vi "realtime track laser dot.vi"() -> ()   [LabVIEW 2015]
doc: "The Low-Level Grab VI acquires images continuously and displays the images in an image control using low-level acquisition VIs. A grab is appropriate for high-speed applications in which you need to process only one image at a time."
uses:
  <vilib>/userdefined/High Color/IMAQdx.ctl
  <vilib>/vision/driver/IMAQdx.llb/IMAQdx Buffer Number Mode.ctl
  <vilib>/vision/driver/NI_Vision_Acquisition_Software.lvlib
  <resource>/objmgr/imaqdx.rc
panel:
  in  "Color of Overlay Text":u32(colorbox)=16448250
  out "time vs iteration":cluster{dbl[], i32[]}(graph)
  out "FPS":i32=42
  out "time (s)":dbl[](array[numeric])=[0.0, 0.04, 0.066, 0.087, 0.114, 0.136, 0.161, 0.184, 0.208, 0.232, 0.257, 0.278, 0.305, 0.328, 0.352, 0.378, 0.399, 0.424, 0.448, 0.473, 0.497, 0.521, 0.545, 0.572, 0.59, 0.614, 0.639, 0.662, 0.686, 0.712, 0.736, 0.761, 0.787, 0.809, 0.834, 0.858, 0.881, 0.907, 0.928, 0.952, 0.978, 1.002, 1.028, 1.049, 1.075, 1.098, 1.124, 1.146, 1.171, 1.197, 1.218, 1.241, 1.267, 1.304, 1.317, 1.336, 1.364, 1.399, 1.411, 1.435, 1.464, 1.49, 1.504, 1.528, 1.566, 1.578, 1.608, 1.629, 1.664, 1.678, 1.709, 1.722, 1.745, 1.768, 1.794, 1.817, 1.842, 1.865, 1.888, 1.913, 1.937, 1.962, 1.987, 2.01, 2.033, 2.058, 2.082, 2.107, 2.132, 2.156, 2.179, 2.203, 2.229, 2.252, 2.278, 2.3, 2.323, 2.348, 2.372, 2.414, 2.426, 2.45, 2.465, 2.489, 2.513, 2.538, 2.562, 2.586, 2.611, 2.634, 2.659, 2.682, 2.708, 2.73, 2.754, 2.778, 2.802, 2.827, 2.85, 2.874, 2.898, 2.922, 2.945, 2.97, 2.995, 3.018, 3.042, 3.066, 3.09, 3.116, 3.139, 3.162, 3.186, 3.211, 3.233, 3.259, 3.282, 3.307, 3.33, 3.355, 3.379, 3.402, 3.427, 3.45, 3.475, 3.499, 3.524, 3.546, 3.571, 3.594, 3.619, 3.643, 3.666, 3.691, 3.715, 3.739, 3.763, 3.787, 3.811, 3.834, 3.86, 3.883, 3.908, 3.931, 3.956, 3.979, 4.003, 4.028, 4.05, 4.076, 4.099, 4.124, 4.147, 4.172, 4.195, 4.219, 4.244, 4.267, 4.292, 4.315, 4.34, 4.363, 4.388, 4.412, 4.437, 4.46, 4.483, 4.51, 4.534, 4.556, 4.582, 4.604, 4.629, 4.653, 4.677, 4.7, 4.725, 4.748, 4.772, 4.796, 4.82, 4.847, 4.868, 4.893, 4.917, 4.941, 4.965, 4.989, 5.013, 5.038, 5.061, 5.085, 5.111, 5.133, 5.159, 5.181, 5.205, 5.229, 5.253, 5.278, 5.301, 5.326, 5.349, 5.374, 5.398, 5.422, 5.445, 5.47, 5.494, 5.518, 5.541, 5.567, 5.59, 5.614, 5.638, 5.662, 5.686, 5.71, 5.734, 5.759, 5.782, 5.806, 5.834, 5.854, 5.879, 5.903, 5.927, 5.95, 5.976, 5.999, 6.023, 6.047, 6.072, 6.095, 6.121, 6.144, 6.167, 6.192, 6.215, 6.24, 6.263, 6.288, 6.312, 6.336, 6.36, 6.383, 6.408, 6.432, 6.457, 6.48, 6.505, 6.529, 6.552, 6.577, 6.6, 6.626, 6.648, 6.673, 6.696, 6.721, 6.746, 6.768, 6.794, 6.816, 6.843, 6.865, 6.89, 6.913, 6.938, 6.962, 6.985, 7.01, 7.034, 7.058, 7.082, 7.106, 7.13, 7.154, 7.178, 7.202, 7.227, 7.25, 7.274, 7.298, 7.322, 7.346, 7.37, 7.395, 7.418, 7.443, 7.466, 7.491, 7.514, 7.539, 7.562, 7.586, 7.611, 7.634, 7.66, 7.682, 7.708, 7.73, 7.756, 7.779, 7.804, 7.827, 7.851, 7.876, 7.899, 7.924, 7.947, 7.971, 7.995, 8.019, 8.043, 8.067, 8.092, 8.116, 8.14, 8.163, 8.187, 8.212, 8.235, 8.26, 8.283, 8.309, 8.331, 8.356, 8.379, 8.404, 8.428, 8.452, 8.477, 8.5, 8.524, 8.551, 8.575, 8.597, 8.621, 8.645, 8.668, 8.694, 8.717, 8.743, 8.765, 8.79, 8.812, 8.837, 8.862, 8.888, 8.913, 8.936, 8.959, 8.986, 9.009, 9.033, 9.057, 9.082, 9.11, 9.128, 9.151, 9.175, 9.202, 9.228, 9.248, 9.271, 9.295, 9.319, 9.344, 9.384, 9.397, 9.415, 9.441, 9.478, 9.491, 9.521, 9.536, 9.563, 9.584, 9.609, 9.631, 9.67, 9.683, 9.706, 9.729, 9.752, 9.776, 9.812, 9.826, 9.849, 9.881, 9.899, 9.922, 9.944, 9.969, 9.993, 10.016, 10.041, 10.066, 10.091, 10.118, 10.14, 10.165, 10.184, 10.21, 10.234, 10.258, 10.294, 10.308, 10.342, 10.355, 10.377, 10.411, 10.424, 10.449, 10.475, 10.507, 10.523, 10.549, 10.58, 10.595, 10.618, 10.646, 10.668, 10.693, 10.716, 10.739, 10.762, 10.8, 10.813, 10.837, 10.862, 10.9, 10.913, 10.931, 10.955, 10.981, 11.007, 11.044, 11.058, 11.076, 11.103, 11.128, 11.15, 11.175, 11.197, 11.23, 11.245, 11.271, 11.294, 11.319, 11.342, 11.37, 11.39, 11.417, 11.438, 11.465, 11.486, 11.512, 11.532, 11.557, 11.581, 11.605, 11.638, 11.654, 11.68, 11.701, 11.727, 11.768, 11.782, 11.797, 11.822, 11.847, 11.873, 11.895, 11.92, 11.943, 11.97, 11.991, 12.016, 12.04, 12.064, 12.099, 12.113, 12.138, 12.159, 12.183, 12.208, 12.234, 12.257, 12.287, 12.309, 12.328, 12.355, 12.375, 12.399, 12.424, 12.451, 12.471, 12.495, 12.519, 12.565, 12.579, 12.592, 12.616, 12.643, 12.661, 12.708, 12.724, 12.736, 12.76, 12.784, 12.81, 12.832, 12.858, 12.88, 12.904, 12.929, 12.952, 12.979, 13.0, 13.025, 13.051, 13.073, 13.098, 13.127, 13.145, 13.169, 13.194, 13.219, 13.241, 13.268, 13.287, 13.313, 13.34, 13.361, 13.388, 13.408, 13.432, 13.459, 13.481, 13.507, 13.529, 13.554, 13.581, 13.602, 13.629, 13.65, 13.676, 13.699, 13.727, 13.747, 13.775, 13.794, 13.819, 13.844, 13.867, 13.893, 13.915, 13.94, 13.965, 13.988, 14.01, 14.04, 14.057, 14.082, 14.108, 14.133, 14.156, 14.18, 14.205, 14.232, 14.252, 14.278, 14.3, 14.326, 14.348, 14.373, 14.397, 14.421, 14.446, 14.468, 14.494, 14.516, 14.541, 14.565, 14.59, 14.611, 14.639, 14.66, 14.688, 14.708, 14.736, 14.757, 14.785, 14.804, 14.83, 14.853, 14.877, 14.902, 14.926, 14.948, 14.974, 14.995, 15.02, 15.046, 15.071, 15.095, 15.121, 15.142, 15.169, 15.191, 15.216, 15.237, 15.263, 15.287, 15.311, 15.333, 15.359, 15.382, 15.409, 15.431, 15.454, 15.48, 15.502, 15.528, 15.55, 15.575, 15.6, 15.621, 15.646, 15.674, 15.696, 15.716, 15.744, 15.768, 15.792, 15.817, 15.84, 15.864, 15.887, 15.912, 15.934, 15.962, 15.984, 16.007, 16.036, 16.056, 16.081, 16.105, 16.129, 16.153, 16.176, 16.2, 16.229, 16.249, 16.273, 16.298, 16.319, 16.348, 16.369, 16.392, 16.419, 16.441, 16.464, 16.492, 16.512, 16.542, 16.56, 16.586, 16.608, 16.633, 16.659, 16.679, 16.704, 16.732, 16.751, 16.777, 16.8, 16.826, 16.848, 16.875, 16.896, 16.92, 16.946, 16.969, 16.995, 17.017, 17.042, 17.063, 17.089, 17.117, 17.139, 17.162, 17.184, 17.211, 17.233, 17.26, 17.281, 17.307, 17.329, 17.357, 17.376, 17.401, 17.426, 17.451, 17.473, 17.499, 17.522, 17.546, 17.573, 17.593, 17.619, 17.642, 17.668, 17.691, 17.713, 17.738, 17.763, 17.792, 17.812, 17.834, 17.861, 17.886, 17.908, 17.933, 17.956, 17.98, 18.005, 18.029, 18.051, 18.078, 18.1, 18.125, 18.15, 18.175, 18.196, 18.221, 18.245, 18.269, 18.293, 18.319, 18.342, 18.366, 18.39, 18.414, 18.438, 18.462, 18.486, 18.511, 18.534, 18.558, 18.583, 18.606, 18.628, 18.657, 18.676, 18.702, 18.724, 18.754, 18.772, 18.797, 18.822, 18.845, 18.867, 18.895, 18.918, 18.941, 18.967, 18.991, 19.013, 19.039, 19.062, 19.085, 19.114, 19.136, 19.158, 19.182, 19.205, 19.229, 19.255, 19.279, 19.303, 19.326, 19.349, 19.376, 19.398, 19.425, 19.444, 19.472, 19.494, 19.52, 19.542, 19.568, 19.591, 19.615, 19.639, 19.663, 19.686, 19.715, 19.733, 19.761, 19.782, 19.809, 19.83, 19.856, 19.877, 19.905, 19.926, 19.951, 19.975, 20.005, 20.023, 20.048, 20.07, 20.096, 20.136, 20.153, 20.168, 20.193, 20.218, 20.24, 20.264, 20.286, 20.322, 20.336, 20.364, 20.385, 20.41, 20.433, 20.456, 20.48, 20.507, 20.529, 20.553, 20.579, 20.601, 20.626, 20.649, 20.673, 20.699, 20.721, 20.745, 20.769, 20.793, 20.824, 20.845, 20.871, 20.887, 20.915, 20.939, 20.962, 20.984, 21.012, 21.037, 21.058, 21.083, 21.106, 21.133, 21.155, 21.181, 21.205, 21.23, 21.252, 21.276, 21.301, 21.324, 21.348, 21.373, 21.396, 21.42, 21.444, 21.47, 21.492, 21.516, 21.54, 21.565, 21.589, 21.612, 21.636, 21.66, 21.687, 21.71, 21.736, 21.758, 21.783, 21.806, 21.832, 21.856, 21.879, 21.903, 21.926, 21.951, 21.975, 22.003, 22.024, 22.047, 22.072, 22.096, 22.123, 22.143, 22.167, 22.188, 22.213, 22.239, 22.266, 22.287, 22.318, 22.335, 22.36, 22.386, 22.405, 22.432, 22.456, 22.479, 22.504, 22.528, 22.552, 22.576, 22.599, 22.621, 22.649, 22.673, 22.696, 22.72, 22.745, 22.77, 22.793, 22.819, 22.841, 22.863, 22.893, 22.921, 22.942, 22.959, 22.984, 23.008, 23.038, 23.057, 23.082, 23.106, 23.13, 23.161] format="%.3f"
  in  "Origin":cluster{"X":i32, "Y":i32}
  out "Y position vs time":cluster{dbl[], i32[]}(graph)
  out "X position vs time":cluster{dbl[], i32[]}(graph)={array[963 elements], [49, 49, 49, 49, 49, 49, 49, 49, 49, 49, 49, 49, 49, 49, 49, 49, 49, 49, 49, 49, 49, 49, 49, 49, 49, 49, 49, 49, 49, 49, 49, 49, 49, 49, 49, 49, 49, 49, 49, 49, 49, 49, 49, 49, 49, 49, 49, 49, 49, 49, 49, 49, 49, 49, 49, 49, 49, 49, 49, 49, 49, 49, 49, 49, 49, 49, 49, 49, 49, 49, 49, 49, 49, 49, 49, 49, 49, 49, 49, 49, 49, 49, 49, 49, 49, 49, 49, 49, 49, 49, 49, 49, 49, 49, 49, 49, 49, 49, 49, 49, 49, 49, 49, 49, 49, 49, 49, 49, 49, 49, 49, 49, 49, 49, 49, 49, 49, 49, 49, 49, 49, 49, 49, 49, 49, 49, 49, 49, 49, 49, 49, 49, 49, 49, 49, 49, 49, 49, 49, 49, 49, 49, 49, 49, 49, 49, 49, 49, 49, 49, 49, 49, 49, 49, 49, 49, 49, 49, 49, 49, 49, 49, 49, 49, 49, 49, 49, 49, 49, 49, 49, 49, 49, 49, 49, 49, 49, 49, 49, 49, 49, 49, 49, 49, 49, 49, 49, 49, 49, 49, 49, 49, 49, 49, 49, 49, 49, 49, 49, 49, 49, 49, 49, 49, 49, 49, 49, 49, 49, 49, 49, 49, 49, 49, 49, 49, 49, 49, 49, 49, 49, 49, 49, 49, 49, 49, 49, 49, 49, 49, 49, 49, 49, 49, 49, 49, 49, 49, 49, 49, 49, 49, 49, 49, 49, 49, 49, 49, 49, 49, 49, 49, 49, 49, 49, 49, 49, 49, 49, 49, 49, 49, 49, 49, 49, 49, 49, 49, 49, 49, 49, 49, 49, 49, 49, 49, 49, 49, 49, 49, 49, 49, 49, 49, 49, 49, 49, 49, 49, 49, 49, 49, 49, 49, 49, 49, 49, 49, 49, 49, 49, 49, 49, 49, 49, 49, 49, 49, 49, 49, 49, 49, 49, 49, 49, 49, 49, 49, 49, 49, 49, 49, 49, 49, 49, 49, 49, 49, 49, 49, 49, 49, 49, 49, 49, 49, 49, 49, 49, 49, 49, 49, 49, 49, 49, 49, 49, 49, 49, 49, 49, 49, 49, 49, 49, 49, 49, 49, 49, 49, 49, 49, 49, 49, 49, 49, 49, 49, 49, 49, 49, 49, 49, 49, 49, 49, 49, 49, 49, 49, 49, 49, 49, 49, 49, 49, 49, 49, 49, 49, 49, 49, 49, 49, 49, 49, 49, 49, 49, 49, 49, 49, 49, 49, 49, 49, 49, 49, 49, 49, 49, 49, 49, 49, 49, 49, 49, 49, 49, 49, 49, 49, 49, 49, 49, 49, 49, 49, 49, 49, 49, 49, 49, 49, 49, 49, 49, 49, 49, 49, 49, 49, 49, 49, 49, 49, 49, 49, 49, 49, 49, 49, 49, 49, 49, 49, 49, 49, 49, 49, 49, 49, 49, 49, 49, 49, 49, 49, 49, 49, 49, 49, 49, 49, 49, 49, 49, 49, 49, 49, 49, 49, 49, 49, 49, 49, 49, 49, 49, 49, 49, 49, 49, 49, 49, 49, 49, 49, 49, 49, 49, 49, 49, 49, 49, 49, 49, 49, 49, 49, 49, 49, 49, 49, 49, 49, 49, 49, 49, 49, 49, 49, 49, 49, 49, 49, 49, 49, 49, 49, 49, 49, 49, 49, 49, 49, 49, 49, 49, 49, 49, 49, 49, 49, 49, 49, 49, 49, 49, 49, 49, 49, 49, 49, 49, 49, 49, 49, 49, 49, 49, 49, 49, 49, 49, 49, 49, 49, 49, 49, 49, 49, 49, 49, 49, 49, 49, 49, 49, 49, 49, 49, 49, 49, 49, 49, 49, 49, 49, 49, 49, 49, 49, 49, 49, 49, 49, 49, 49, 49, 49, 49, 49, 49, 49, 49, 49, 49, 49, 49, 49, 49, 49, 49, 49, 49, 49, 49, 49, 49, 49, 49, 49, 49, 49, 49, 49, 49, 49, 49, 49, 49, 49, 49, 49, 49, 49, 49, 49, 49, 49, 49, 49, 49, 49, 49, 49, 49, 49, 49, 49, 49, 49, 49, 49, 49, 49, 49, 49, 49, 49, 49, 49, 49, 49, 49, 49, 49, 49, 49, 49, 49, 49, 49, 49, 49, 49, 49, 49, 49, 49, 49, 49, 49, 49, 49, 49, 49, 49, 49, 49, 49, 49, 49, 49, 49, 49, 49, 49, 49, 49, 49, 49, 49, 49, 49, 49, 49, 49, 49, 49, 49, 49, 49, 49, 49, 49, 49, 49, 49, 49, 49, 49, 49, 49, 49, 49, 49, 49, 49, 49, 49, 49, 49, 49, 49, 49, 49, 49, 49, 49, 49, 49, 49, 49, 49, 49, 49, 49, 49, 49, 49, 49, 49, 49, 49, 49, 49, 49, 49, 49, 49, 49, 49, 49, 49, 49, 49, 49, 49, 49, 49, 49, 49, 49, 49, 49, 49, 49, 49, 49, 49, 49, 49, 49, 49, 49, 49, 49, 49, 49, 49, 49, 49, 49, 49, 49, 49, 49, 49, 49, 49, 49, 49, 49, 49, 49, 49, 49, 49, 49, 49, 49, 49, 49, 49, 49, 49, 49, 49, 49, 49, 49, 49, 49, 49, 49, 49, 49, 49, 49, 49, 49, 49, 49, 49, 49, 49, 49, 49, 49, 49, 49, 49, 49, 49, 49, 49, 49, 49, 49, 49, 49, 49, 49, 49, 49, 49, 49, 49, 49, 49, 49, 49, 49, 49, 49, 49, 49, 49, 49, 49, 49, 49, 49, 49, 49, 49, 49, 49, 49, 49, 49, 49, 49, 49, 49, 49, 49, 49, 49, 49, 49, 49, 49, 49, 49, 49, 49, 49, 49, 49, 49, 49, 49, 49, 49, 49, 49, 49, 49, 49, 49, 49, 49, 49, 49, 49, 49, 49, 49, 49, 49, 49, 49, 49, 49, 49, 49, 49, 49, 49, 49, 49, 49, 49, 49, 49, 49, 49, 49, 49, 49, 49, 49, 49, 49, 49, 49, 49, 49, 49, 49, 49, 49, 49, 49, 49, 49, 49, 49, 49, 49]}
  in  "threshhold":i32=221
  out "found\nedge\nin ROI":bool[](array[boolean])
  in  "image row min":i32=50
  in  "image row max":i32=1150
  in  "image col min":i32=50
  in  "image col max":i32=1900
  out "X positions\n(image \ncoordinates)":i32[](array[numeric])=[49, 49, 49, 49, 49, 49, 49, 49, 49, 49, 49, 49, 49, 49, 49, 49, 49, 49, 49, 49, 49, 49, 49, 49, 49, 49, 49, 49, 49, 49, 49, 49, 49, 49, 49, 49, 49, 49, 49, 49, 49, 49, 49, 49, 49, 49, 49, 49, 49, 49, 49, 49, 49, 49, 49, 49, 49, 49, 49, 49, 49, 49, 49, 49, 49, 49, 49, 49, 49, 49, 49, 49, 49, 49, 49, 49, 49, 49, 49, 49, 49, 49, 49, 49, 49, 49, 49, 49, 49, 49, 49, 49, 49, 49, 49, 49, 49, 49, 49, 49, 49, 49, 49, 49, 49, 49, 49, 49, 49, 49, 49, 49, 49, 49, 49, 49, 49, 49, 49, 49, 49, 49, 49, 49, 49, 49, 49, 49, 49, 49, 49, 49, 49, 49, 49, 49, 49, 49, 49, 49, 49, 49, 49, 49, 49, 49, 49, 49, 49, 49, 49, 49, 49, 49, 49, 49, 49, 49, 49, 49, 49, 49, 49, 49, 49, 49, 49, 49, 49, 49, 49, 49, 49, 49, 49, 49, 49, 49, 49, 49, 49, 49, 49, 49, 49, 49, 49, 49, 49, 49, 49, 49, 49, 49, 49, 49, 49, 49, 49, 49, 49, 49, 49, 49, 49, 49, 49, 49, 49, 49, 49, 49, 49, 49, 49, 49, 49, 49, 49, 49, 49, 49, 49, 49, 49, 49, 49, 49, 49, 49, 49, 49, 49, 49, 49, 49, 49, 49, 49, 49, 49, 49, 49, 49, 49, 49, 49, 49, 49, 49, 49, 49, 49, 49, 49, 49, 49, 49, 49, 49, 49, 49, 49, 49, 49, 49, 49, 49, 49, 49, 49, 49, 49, 49, 49, 49, 49, 49, 49, 49, 49, 49, 49, 49, 49, 49, 49, 49, 49, 49, 49, 49, 49, 49, 49, 49, 49, 49, 49, 49, 49, 49, 49, 49, 49, 49, 49, 49, 49, 49, 49, 49, 49, 49, 49, 49, 49, 49, 49, 49, 49, 49, 49, 49, 49, 49, 49, 49, 49, 49, 49, 49, 49, 49, 49, 49, 49, 49, 49, 49, 49, 49, 49, 49, 49, 49, 49, 49, 49, 49, 49, 49, 49, 49, 49, 49, 49, 49, 49, 49, 49, 49, 49, 49, 49, 49, 49, 49, 49, 49, 49, 49, 49, 49, 49, 49, 49, 49, 49, 49, 49, 49, 49, 49, 49, 49, 49, 49, 49, 49, 49, 49, 49, 49, 49, 49, 49, 49, 49, 49, 49, 49, 49, 49, 49, 49, 49, 49, 49, 49, 49, 49, 49, 49, 49, 49, 49, 49, 49, 49, 49, 49, 49, 49, 49, 49, 49, 49, 49, 49, 49, 49, 49, 49, 49, 49, 49, 49, 49, 49, 49, 49, 49, 49, 49, 49, 49, 49, 49, 49, 49, 49, 49, 49, 49, 49, 49, 49, 49, 49, 49, 49, 49, 49, 49, 49, 49, 49, 49, 49, 49, 49, 49, 49, 49, 49, 49, 49, 49, 49, 49, 49, 49, 49, 49, 49, 49, 49, 49, 49, 49, 49, 49, 49, 49, 49, 49, 49, 49, 49, 49, 49, 49, 49, 49, 49, 49, 49, 49, 49, 49, 49, 49, 49, 49, 49, 49, 49, 49, 49, 49, 49, 49, 49, 49, 49, 49, 49, 49, 49, 49, 49, 49, 49, 49, 49, 49, 49, 49, 49, 49, 49, 49, 49, 49, 49, 49, 49, 49, 49, 49, 49, 49, 49, 49, 49, 49, 49, 49, 49, 49, 49, 49, 49, 49, 49, 49, 49, 49, 49, 49, 49, 49, 49, 49, 49, 49, 49, 49, 49, 49, 49, 49, 49, 49, 49, 49, 49, 49, 49, 49, 49, 49, 49, 49, 49, 49, 49, 49, 49, 49, 49, 49, 49, 49, 49, 49, 49, 49, 49, 49, 49, 49, 49, 49, 49, 49, 49, 49, 49, 49, 49, 49, 49, 49, 49, 49, 49, 49, 49, 49, 49, 49, 49, 49, 49, 49, 49, 49, 49, 49, 49, 49, 49, 49, 49, 49, 49, 49, 49, 49, 49, 49, 49, 49, 49, 49, 49, 49, 49, 49, 49, 49, 49, 49, 49, 49, 49, 49, 49, 49, 49, 49, 49, 49, 49, 49, 49, 49, 49, 49, 49, 49, 49, 49, 49, 49, 49, 49, 49, 49, 49, 49, 49, 49, 49, 49, 49, 49, 49, 49, 49, 49, 49, 49, 49, 49, 49, 49, 49, 49, 49, 49, 49, 49, 49, 49, 49, 49, 49, 49, 49, 49, 49, 49, 49, 49, 49, 49, 49, 49, 49, 49, 49, 49, 49, 49, 49, 49, 49, 49, 49, 49, 49, 49, 49, 49, 49, 49, 49, 49, 49, 49, 49, 49, 49, 49, 49, 49, 49, 49, 49, 49, 49, 49, 49, 49, 49, 49, 49, 49, 49, 49, 49, 49, 49, 49, 49, 49, 49, 49, 49, 49, 49, 49, 49, 49, 49, 49, 49, 49, 49, 49, 49, 49, 49, 49, 49, 49, 49, 49, 49, 49, 49, 49, 49, 49, 49, 49, 49, 49, 49, 49, 49, 49, 49, 49, 49, 49, 49, 49, 49, 49, 49, 49, 49, 49, 49, 49, 49, 49, 49, 49, 49, 49, 49, 49, 49, 49, 49, 49, 49, 49, 49, 49, 49, 49, 49, 49, 49, 49, 49, 49, 49, 49, 49, 49, 49, 49, 49, 49, 49, 49, 49, 49, 49, 49, 49, 49, 49, 49, 49, 49, 49, 49, 49, 49, 49, 49, 49, 49, 49, 49, 49, 49, 49, 49, 49, 49, 49, 49, 49, 49, 49, 49, 49, 49, 49, 49, 49, 49, 49, 49, 49, 49, 49, 49, 49, 49, 49, 49, 49, 49, 49, 49, 49, 49, 49, 49, 49, 49, 49, 49, 49, 49, 49, 49, 49, 49, 49, 49, 49, 49, 49, 49, 49, 49, 49, 49, 49, 49, 49, 49, 49, 49, 49, 49, 49, 49, 49, 49, 49, 49, 49, 49, 49, 49, 49, 49, 49, 49, 49, 49]
  out "Y positions \n(image \ncoordinates)":i32[](array[numeric])=[433, 433, 432, 433, 433, 433, 433, 433, 433, 433, 433, 433, 433, 433, 433, 433, 433, 433, 433, 433, 432, 433, 433, 433, 432, 433, 433, 433, 434, 433, 433, 434, 433, 433, 433, 434, 433, 433, 433, 433, 433, 433, 433, 433, 433, 434, 433, 433, 433, 433, 433, 434, 433, 433, 433, 433, 433, 433, 433, 433, 433, 433, 433, 433, 433, 433, 433, 433, 433, 433, 433, 433, 432, 433, 433, 433, 432, 433, 433, 433, 433, 433, 434, 433, 433, 432, 433, 433, 433, 433, 433, 433, 433, 433, 433, 435, 433, 432, 433, 433, 435, 433, 433, 433, 433, 433, 433, 433, 433, 433, 434, 433, 433, 433, 433, 433, 433, 433, 433, 433, 433, 433, 433, 433, 433, 433, 432, 433, 433, 433, 433, 433, 433, 433, 433, 433, 434, 433, 433, 433, 433, 433, 433, 433, 433, 433, 433, 433, 433, 433, 433, 433, 433, 433, 433, 433, 433, 432, 433, 433, 434, 433, 433, 433, 433, 433, 433, 433, 434, 433, 432, 433, 433, 433, 433, 433, 433, 433, 433, 433, 433, 433, 433, 433, 433, 433, 433, 433, 433, 433, 433, 433, 433, 433, 433, 433, 432, 433, 432, 433, 432, 433, 433, 434, 433, 433, 434, 433, 434, 433, 433, 433, 432, 433, 434, 433, 433, 433, 433, 434, 433, 433, 433, 433, 433, 432, 433, 433, 433, 433, 433, 433, 433, 433, 433, 433, 433, 433, 433, 433, 433, 433, 433, 433, 433, 433, 433, 433, 434, 433, 433, 433, 433, 433, 433, 432, 433, 433, 433, 433, 433, 433, 433, 433, 434, 434, 433, 432, 433, 433, 433, 433, 432, 433, 433, 433, 432, 433, 433, 433, 433, 434, 433, 433, 434, 433, 433, 433, 433, 433, 433, 433, 433, 433, 433, 433, 433, 433, 433, 433, 433, 433, 433, 433, 434, 433, 432, 434, 433, 432, 433, 432, 433, 433, 433, 434, 433, 434, 433, 434, 433, 433, 433, 433, 432, 433, 433, 433, 433, 433, 433, 433, 434, 433, 433, 433, 433, 433, 434, 432, 433, 434, 433, 433, 433, 433, 433, 433, 433, 433, 433, 433, 433, 433, 433, 433, 433, 433, 432, 433, 434, 433, 433, 433, 433, 433, 433, 433, 433, 433, 433, 434, 433, 433, 433, 433, 433, 432, 433, 433, 432, 434, 433, 434, 433, 433, 432, 433, 433, 433, 433, 433, 433, 434, 433, 433, 433, 433, 433, 433, 434, 433, 433, 435, 433, 433, 433, 433, 433, 433, 433, 433, 433, 433, 432, 433, 432, 433, 433, 433, 433, 432, 433, 433, 433, 433, 433, 433, 433, 433, 433, 433, 433, 433, 433, 433, 433, 433, 433, 433, 433, 434, 433, 433, 433, 433, 433, 433, 432, 434, 433, 433, 433, 433, 434, 433, 433, 433, 432, 433, 433, 433, 433, 433, 433, 433, 434, 433, 433, 432, 433, 433, 433, 433, 433, 432, 433, 433, 433, 433, 433, 433, 433, 433, 433, 433, 433, 432, 433, 433, 433, 433, 433, 433, 433, 433, 434, 433, 432, 433, 433, 433, 433, 433, 432, 433, 434, 433, 433, 433, 433, 433, 433, 433, 433, 433, 433, 433, 433, 433, 433, 433, 433, 433, 433, 433, 432, 433, 433, 433, 432, 433, 433, 433, 433, 433, 433, 434, 433, 432, 433, 433, 433, 433, 433, 433, 433, 433, 433, 433, 433, 433, 433, 433, 433, 433, 433, 433, 434, 433, 433, 433, 433, 434, 433, 433, 433, 433, 433, 433, 433, 433, 433, 434, 434, 433, 434, 433, 433, 433, 433, 433, 433, 433, 434, 434, 433, 433, 433, 433, 433, 434, 433, 433, 433, 433, 433, 433, 433, 433, 433, 433, 433, 433, 433, 433, 433, 433, 433, 433, 433, 433, 433, 433, 433, 433, 433, 433, 432, 433, 433, 433, 432, 433, 433, 433, 433, 433, 433, 433, 433, 432, 433, 433, 433, 433, 434, 433, 433, 433, 433, 433, 433, 433, 433, 433, 434, 433, 433, 433, 433, 433, 433, 433, 433, 433, 433, 433, 433, 433, 433, 433, 432, 433, 433, 433, 433, 433, 433, 433, 433, 433, 433, 433, 433, 433, 433, 434, 434, 433, 433, 433, 433, 433, 433, 434, 433, 433, 433, 433, 433, 433, 432, 433, 433, 433, 433, 433, 433, 433, 433, 433, 433, 433, 433, 433, 433, 434, 434, 433, 433, 433, 433, 433, 432, 433, 433, 433, 433, 433, 433, 434, 433, 433, 433, 433, 433, 433, 433, 433, 433, 433, 433, 433, 433, 433, 433, 433, 433, 433, 432, 434, 433, 433, 433, 433, 433, 433, 433, 433, 433, 433, 433, 433, 433, 433, 433, 433, 433, 433, 433, 433, 433, 433, 432, 433, 433, 433, 433, 433, 433, 433, 433, 433, 433, 433, 433, 433, 433, 434, 433, 433, 433, 433, 433, 433, 433, 433, 433, 434, 433, 433, 434, 433, 433, 433, 434, 434, 433, 434, 433, 433, 434, 433, 433, 433, 433, 434, 433, 433, 433, 433, 433, 433, 433, 433, 433, 433, 433, 433, 433, 433, 433, 433, 433, 433, 433, 433, 433, 433, 433, 433, 433, 433, 433, 433, 433, 433, 433, 433, 433, 433, 433, 433, 433, 433, 433, 433, 433, 433, 433, 433, 433, 433, 433, 433, 433, 433, 433, 433, 433, 433, 433, 433, 433, 433, 433, 432, 433, 433, 433, 433, 433, 433, 433, 433, 433, 434, 434, 434, 432, 433, 433, 433, 432, 433, 433, 433, 433, 433, 433, 434, 433, 433, 433, 433, 433, 433, 433, 433, 433, 433, 433, 433, 433, 433, 433, 433, 433, 433, 434, 433, 432, 433, 433, 433, 433, 434, 433, 433, 433, 433, 433, 433, 433, 433, 433, 433, 433, 433, 434, 433, 433, 433, 433, 433, 433, 433, 433, 433, 434, 433, 434, 433, 433, 433, 434, 433, 433, 433, 433, 432, 434, 433, 433, 433, 433, 433, 433, 433, 434, 434, 433]
  out "LIVE":bool
  in  "stop":bool
  out "Backlog":i32(slide) scale=0.0..50.0
  in  "IMAQdx Device":T1="cam0"
  in  "Buffers":u32=50
  out "Image":T2(plugin-control)
  # "INSTRUCTIONS\n\nThis program finds the \ndarkest searching from\nright to left in an image.\nUsed to find trailing\nedge position of a\nswimming fish. Dark fish\non a light background.\n\nCan also be modified to \nfind lightest."
  # "issues\n\nHow do we know if frames \nare dropped?\n\nProbably will need to save data\nin sections to an open file\n\nCould have a sliding ROI based\non previous trailing edge position\n\nCould process each data chunk\nseparately to avoid frame dropping\nissues.  I.e. if you write every 1000\npoints, then in post processing only\nprocess 1000 at a time."
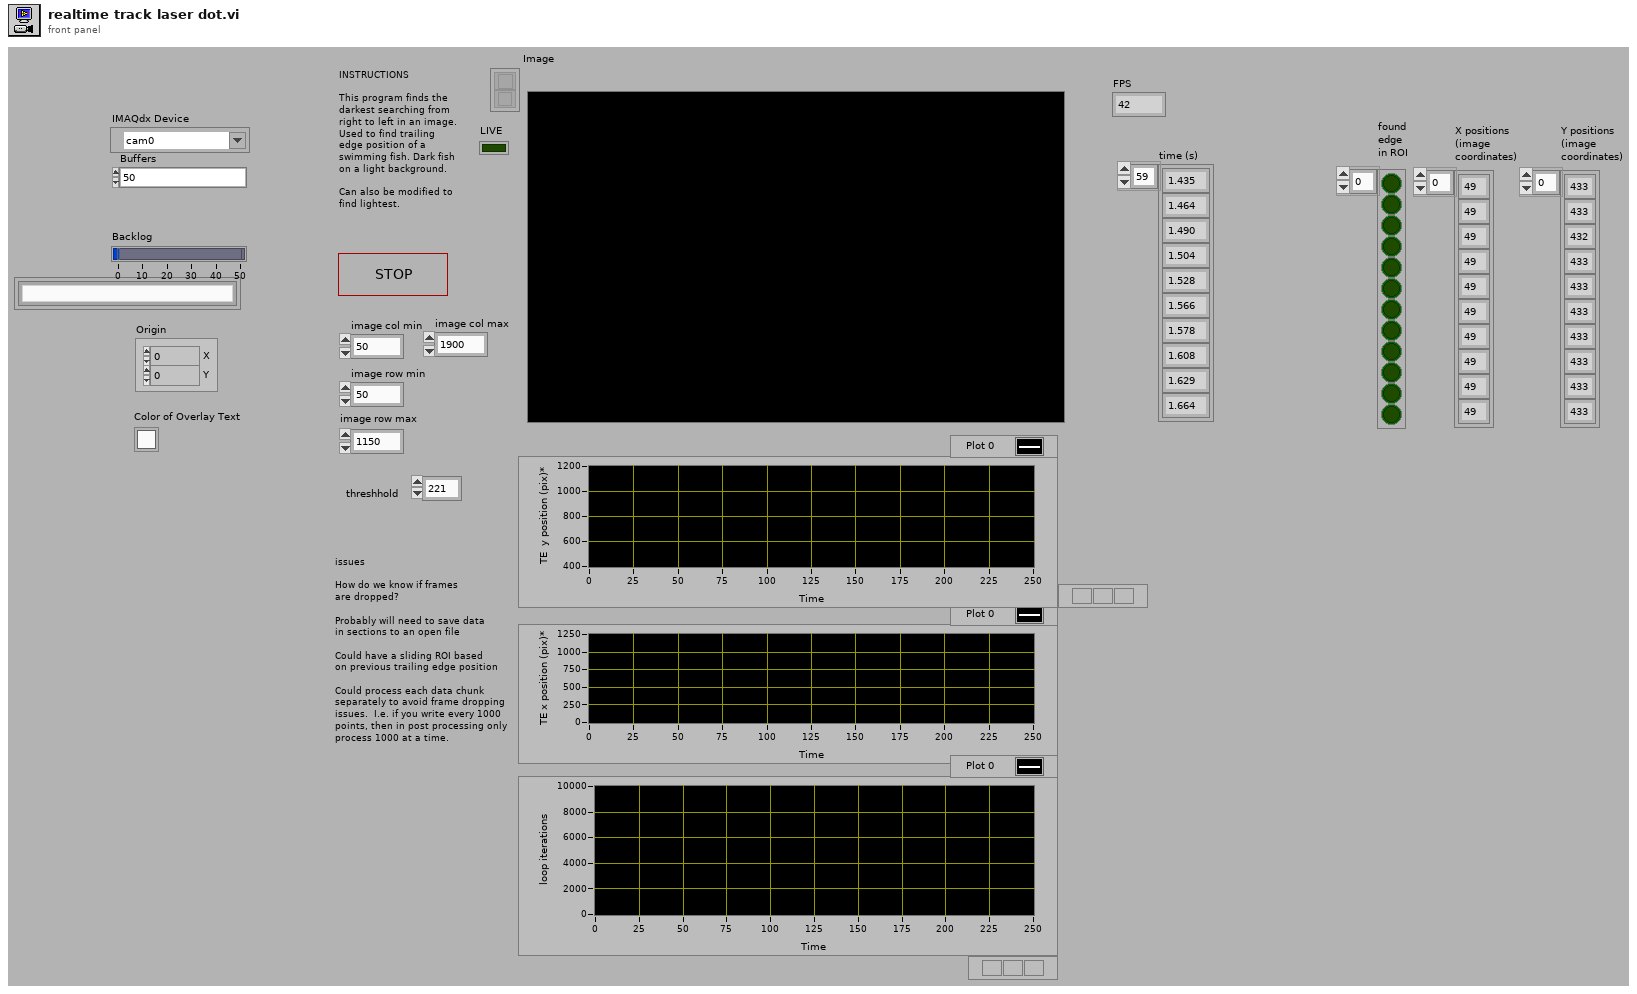
[diagram p1: front panel]
types:
  T1 = typedef "IMAQdx.ctl" = refnum<k21>
  T2 = typedef "IMAQ Image.ctl" = refnum<image>
  T3 = typedef "NI_Vision_Acquisition_Software.lvlib/IMAQdx Buffer Number Mode.ctl" = enum32{"Next", "Last", "Buffer Number", "Every", "Last New"}
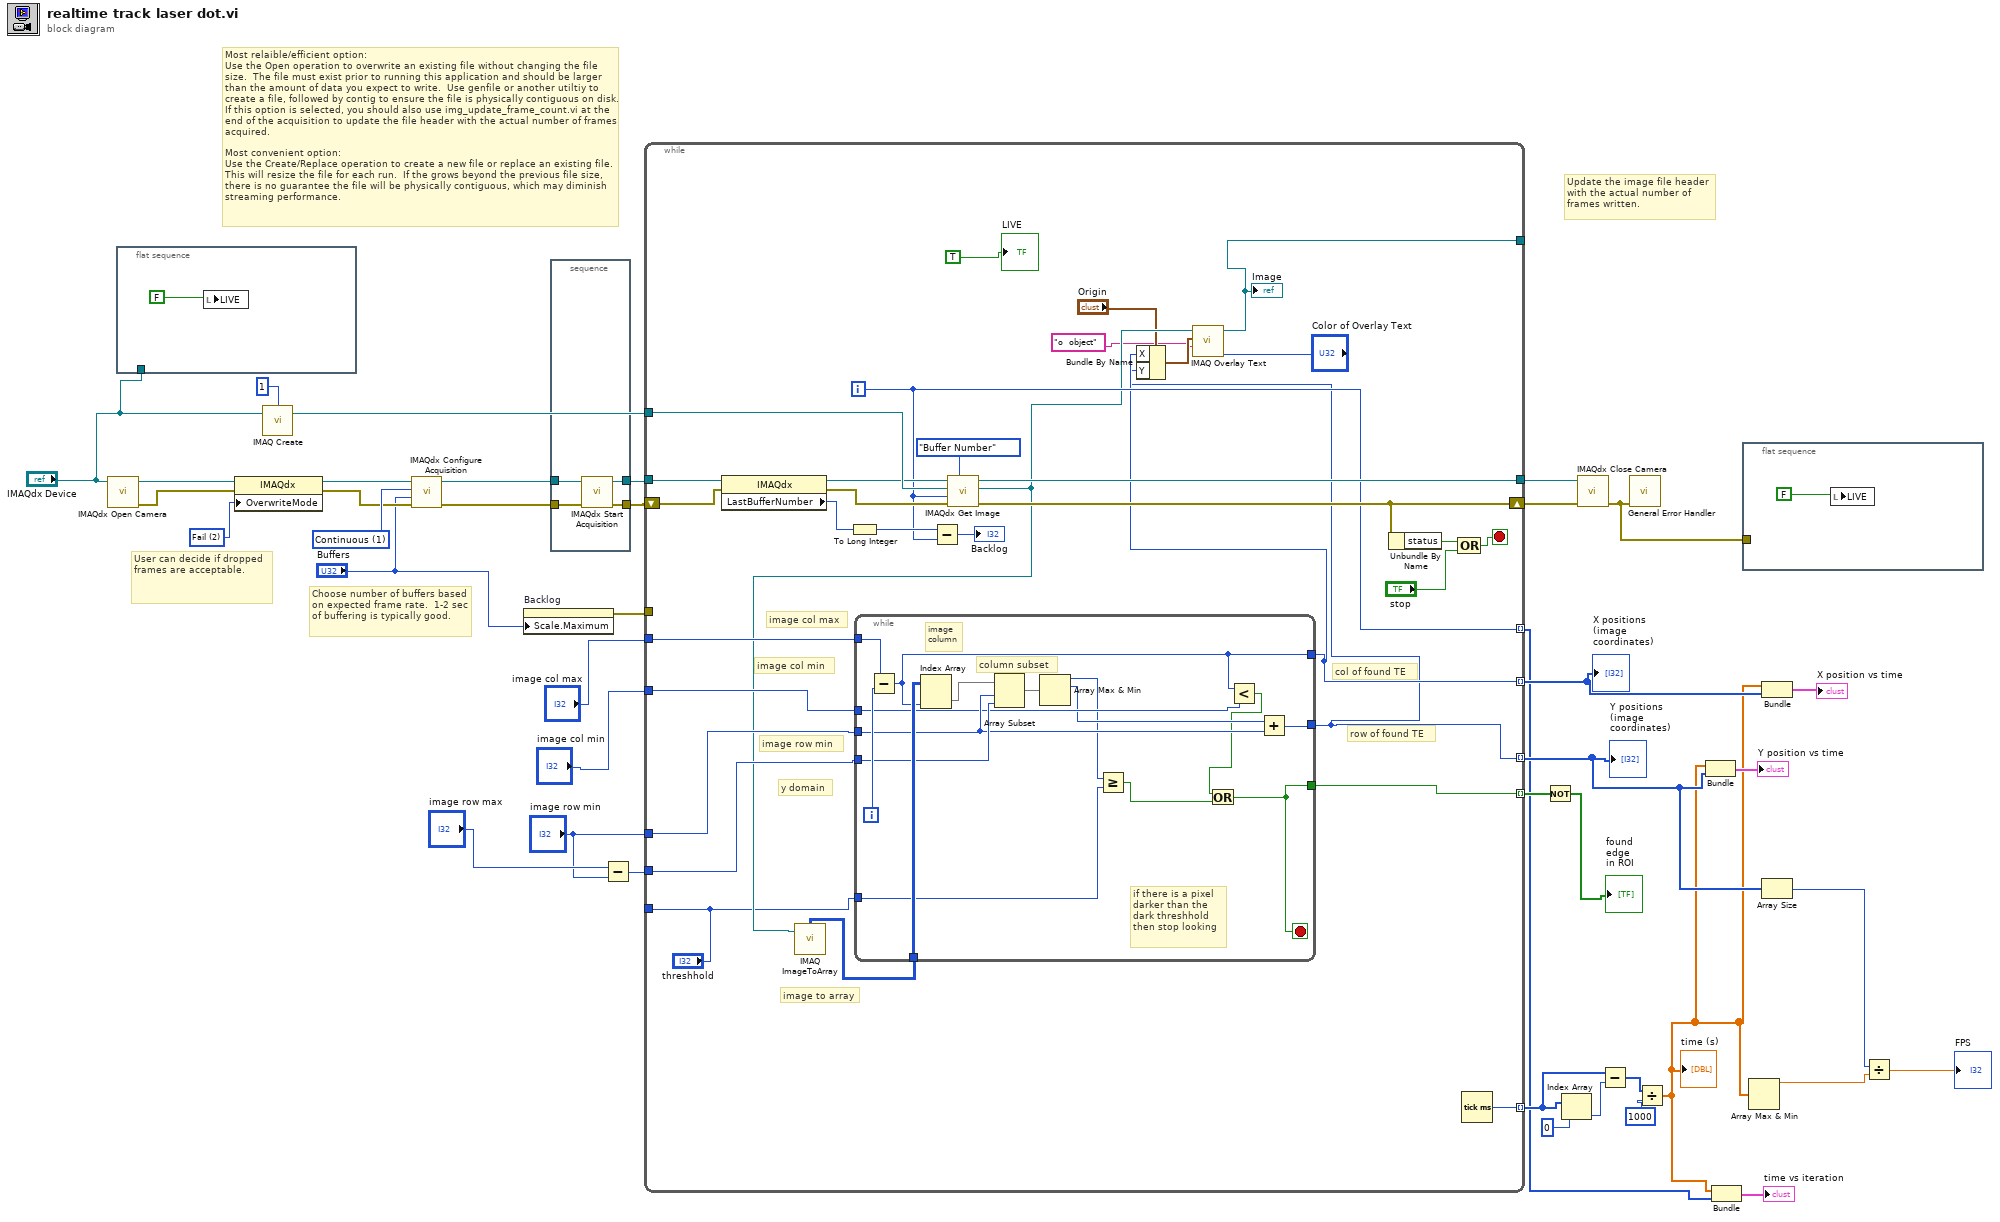
[diagram p0: block diagram]
diagram:
  w33 = u32 2 items=["Get Oldest"=0, "Fail"=2, "Get Newest"=3] ("OverwriteMode")
  w39 = u32 1 items=["One Shot", "Continuous"] ("Continuous ?")
  # "Update the image file header with the actual number of frames written."
  # "Choose number of buffers based on expected frame rate.  1-2 sec of buffering is typically good."
  # "User can decide if dropped frames are acceptable."
  # "Most relaible/efficient option:\nUse the Open operation to overwrite an existing file without changing the file size.  The file must exist prior to running this application and should be larger than the amount of data you expect to write.  Use genfile or another utiltiy to create a file, followed by contig to ensure the file is physically contiguous on disk.  If this option is selected, you should also use img_update_frame_count.vi at the end of the acquisition to update the file header with the actual number of frames acquired. \n\nMost convenient option:\nUse the Create/Replace operation to create a new file or replace an existing file. This will resize the file for each run.  If the grows beyond the previous file size, there is no guarantee the file will be physically contiguous, which may diminish streaming performance."
  n1 = call <vilib>:"IMAQdx Open Camera.vi"("Session In"="IMAQdx Device") -> ("error out"=w29:errorcluster, "Session Out"=w28:T1)  [unwired: 2 in, 7 out]
  n2 = flat-sequence {
    tunnel: "IMAQdx Device" -> [_]
    frame #0 {
      n3 = local write "LIVE"(FALSE) -> ()
    }
  }
  n4 = property class="IMAQdx"(reference=w28, error in=w29, "OverwriteMode"=w33) -> (reference out=w31:T1, error out=w30:errorcluster)
  n5 = call "IMAQ Create"("Border Size"=1, "Image Name"="IMAQdx Device") -> ("New Image"=w40:T2)  [unwired: 2 in, 2 out]
  n6 = call <vilib>:"IMAQdx Configure Acquisition.vi"("error in"=w30, "Number of Buffers"="Buffers", "Continuous?"=w39, "Session In"=w31) -> ("error out"=w25:errorcluster, "Session Out"=w32:T1)  [unwired: 6 out]
  n7 = property on="Backlog" class="Slide (strict)"("Scale.Maximum"="Buffers") -> (error out=w27:errorcluster)  [unwired: 2 in, 1 out]
  n8 = stacked-sequence {
    tunnel: [w45] -> w38
    tunnel: [w44] -> w37
    tunnel: w32 -> [w43]
    tunnel: w25 -> [w42]
    frame #0 {
      n9 = call <vilib>:"IMAQdx Start Acquisition.vi"("error in"=w42, "Session In"=w43) -> ("error out"=w45:errorcluster, "Session Out"=w44:T1)  [unwired: 8 out]
    }
  }
  n10 = Subtract(x="image row max", y="image row min") -> (x-y=w18:i32)
  n11 = while {
    tunnel: [w72] -> w35
    tunnel: w37 -> [w75]
    tunnel: w40 -> [w73]
    tunnel: [w54] -> _
    shift-right: [w71] -> w34
    shift-left: w38 -> [w74]
    tunnel: w27 -> [_]
    tunnel: "image col max" -> [w61]
    tunnel: "image col min" -> [w60]
    tunnel: "image row min" -> [w59]
    tunnel: w18 -> [w58]
    tunnel: ["threshhold"] -> _
    tunnel: [w52] -> w15 mode=indexing
    tunnel: [w51] -> w8 mode=indexing
    tunnel: [w57] -> w17 mode=indexing
    tunnel: [w56] -> w2 mode=indexing
    tunnel: [w48] -> w10 mode=indexing
    i -> [w56]
    stop <- w77 stop-if-true
    # "image col min"
    # "image col max"
    # "image row min"
    # "row of found TE"
    # "col of found TE"
    # "y domain"
    # "image to array"
    n12 = property class="IMAQdx"(reference=w75, error in=w74) -> (reference out=w68:T1, error out=w69:errorcluster, "LastBufferNumber"=w65:u32)
    n13 = To Long Integer(number=w65) -> (32bit integer=w64:i32)
    n14 = Subtract(x=w64, y=w56) -> (x-y=→"Backlog":i32)
    n15 = call <vilib>:"IMAQdx Get Image.vi"("Buffer Number Mode (Next)"=IMAQdx_Buffer_Number_Mode."Buffer Number", "error in"=w69, "Buffer Number In"=w56, "Image In"=w73, "Session In"=w68) -> ("error out"=w71:errorcluster, "Image Out"=w55:T2, "Session Out"=w72:T1)  [unwired: 1 in, 3 out]
    n16 = call "IMAQ ImageToArray"("Image"=w55) -> ("Image Pixels (U8)"=w62:u8[][])  [unwired: 2 in, 5 out]
    n17 = while {
      tunnel: w59 -> [w86]
      tunnel: [w84] -> w52
      tunnel: [w87] -> w51
      tunnel: w58 -> [w89]
      tunnel: w62 -> [w91]
      tunnel: w61 -> [w93]
      tunnel: w60 -> [w85]
      tunnel: [w80] -> w57
      tunnel: "threshhold" -> [w82]
      i -> [w92]
      stop <- w80 stop-if-true
      # "if there is a pixel\ndarker than the\ndark threshhold\nthen stop looking"
      # "column subset"
      # "image\ncolumn"
      n18 = Subtract(x=w93, y=w92) -> (x-y=w84:i32)
      n19 = Index Array(array=w91, index (col)=w84) -> (element=w90:u8[])  [unwired: 1 in]
      n20 = Array Subset(array=w90, index=w86, length=w89) -> (w88:u8[])
      n21 = Array Max & Min(array=w88) -> (max value=w81:u8, max index (indices)=w83:i32)  [unwired: 2 out]
      n22 = Greater Or Equal?(x=w81, y=w82) -> (x >= y?=w78:bool)
      n23 = Less?(x=w84, y=w85) -> (x < y?=w79:bool)
      n24 = Or(x=w79, y=w78) -> (x .or. y?=w80:bool)
      n25 = Add(x=w83, y=w86) -> (x+y=w87:i32)
    }
    n26 = Bundle By Name(cluster="Origin", "X"=w52, "Y"=w51) -> (w50:cluster{"X":i32, "Y":i32})
    n27 = call "IMAQ Overlay Text"("Text Color (black)"="Color of Overlay Text", "String"="o  object", "Origin"=w50, "Image"=w55) -> ("Image Out"=w54:T2)  [unwired: 4 in, 3 out]
    "Image" <- w54
    n28 = Unbundle By Name(w71) -> ("status"=w76:bool)
    n29 = Compound Arithmetic op=OR(w76, "stop") -> (w77:bool)
    n30 = Tick Count (ms)() -> (millisecond timer value=w48:u32)
    "LIVE" <- TRUE
  }
  "X positions\n(image \ncoordinates)" <- w15
  "Y positions \n(image \ncoordinates)" <- w8
  n31 = Not(x=w17) -> (.not. x?=→"found\nedge\nin ROI":bool[])
  n32 = Index Array(array=w10, index=0) -> (element=w11:u32)
  n33 = call <vilib>:"IMAQdx Close Camera.vi"("error in"=w34, "Session In"=w35) -> ("error out"=w24:errorcluster)  [unwired: 9 out]
  n34 = Subtract(x=w10, y=w11) -> (x-y=w3:u32[])
  n35 = call <vilib>:"General Error Handler.vi"("error in (no error)"=w24) -> ()  [unwired: 2 in, 13 out]
  n36 = Divide(x=w3, y=1000) -> (x/y=w1:dbl[])
  "time (s)" <- w1
  n37 = Bundle(w1, w8) -> (→"Y position vs time":cluster{dbl[], i32[]})  [unwired: 1 out]
  n38 = Bundle(w1, w2) -> (→"time vs iteration":cluster{dbl[], i32[]})  [unwired: 1 out]
  n39 = flat-sequence {
    tunnel: w24 -> [_]
    frame #0 {
      n40 = local write "LIVE"(FALSE) -> ()
    }
  }
  n41 = Array Max & Min(array=w1) -> (max value=w9:dbl)  [unwired: 3 out]
  n42 = Bundle(w1, w15) -> (→"X position vs time":cluster{dbl[], i32[]})  [unwired: 1 out]
  n43 = Array Size(array=w8) -> (size(s)=w7:i32)
  n44 = Divide(x=w7, y=w9) -> (x/y=→"FPS":dbl)
